vi "ProjectConnect.vi"(8 "error in (no error)":errorcluster) -> (0 "error out":errorcluster, 3 "Project Ref out":T1)   [LabVIEW 2015, in "ni-veristand-steps-runtime-lib.lvlib"]
uses:
  ni-veristand-steps-runtime-lib.lvlib
  <vilib>/NI Veristand/Execution/Project/Project Ref.ctl
  NationalInstruments.VeriStand.ClientAPI
  <vilib>/NI Veristand/Execution/Project/NI_VS Project ExecutionAPI.lvlib
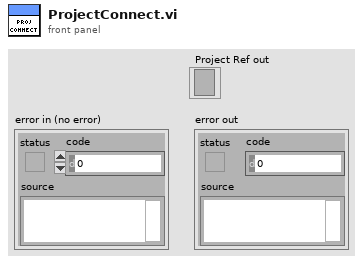
[diagram p1: front panel]
types:
  T1 = typedef "NI_VS Project ExecutionAPI.lvlib/Project Ref.ctl" = refnum<k24>
  T2 = typedef "ni-veristand-steps-runtime-lib.lvlib/VeriStand dotNet References.ctl" = cluster{"ModelManager":T3, "AlarmManager":T4, "ChannelFault":T5, "WorkspaceManager":T6, "Project Ref":T1}
  T3 = typedef "NI_VS ModelManager ExecutionAPI.lvlib/ModelManagerAPI.ctl" = refnum<k24>
  T4 = typedef "NI_VS AlarmManager ExecutionAPI.lvlib/AlarmManagerAPI.ctl" = refnum<k24>
  T5 = typedef "NI_VS ChannelFault ExecutionAPI.lvlib/ChannelFaultAPI.ctl" = refnum<k24>
  T6 = typedef "NI_VS Workspace ExecutionAPI.lvlib/WorkspaceAPI.ctl" = refnum<k24>
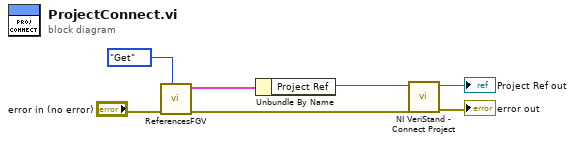
[diagram p0: block diagram]
diagram:
  n1 = call "ReferencesFGV.vi"("Get/Set"=enum16{"Get", "Set"}."Get", "error in (no error)"="error in (no error)") -> ("error out"=w2:errorcluster, "VeriStand dotNET Refs out"=w5:T2)  [unwired: 8 in]
  n2 = Unbundle By Name(w5) -> ("Project Ref"=w3:T1)
  n3 = call <vilib>:"NI VeriStand - Connect Project.vi"("error in (no error)"=w2, "Project Ref in"=w3) -> ("error out"=→"error out":errorcluster, "Project Ref out"=→"Project Ref out":T1)  [unwired: 8 in]
